vi "Read From Spreadsheet File (string)-Mod.vi"(0 "file path (dialog if empty)":path, 1 "format (%s)":string="%s", 5 "number of rows (all:-1)":i32=-1, 7 "max characters/row  (no limit:0)":i32, 9 "start of read offset (chars.:0)":i32, 11 "error in":errorcluster, 12 "transpose (no:F)":bool, 14 "delimiter (\\t)":string="\t") -> (3 "new file path (Not A Path if cancelled)":path, 4 "all rows":string[][](array[string]), 6 "first row":string[](array[string]), 8 "EOF?":bool, 10 "mark after read (chars.)":i32, 15 "error out":errorcluster)   [LabVIEW 2013]
doc: "Reads a specified number of lines or rows from a numeric text file beginning at a specified character offset and converts the data to a 2D, double-precision array of numbers, strings, or integers. You must manually select the polymorphic instance you want to use."
panel:
  in  "type (empty)":string[][](array[string])
  # "row\ncolumn"
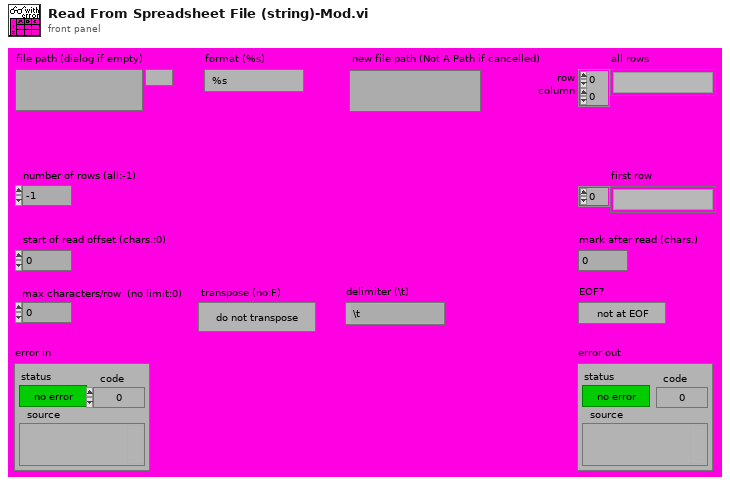
[diagram p1: front panel]
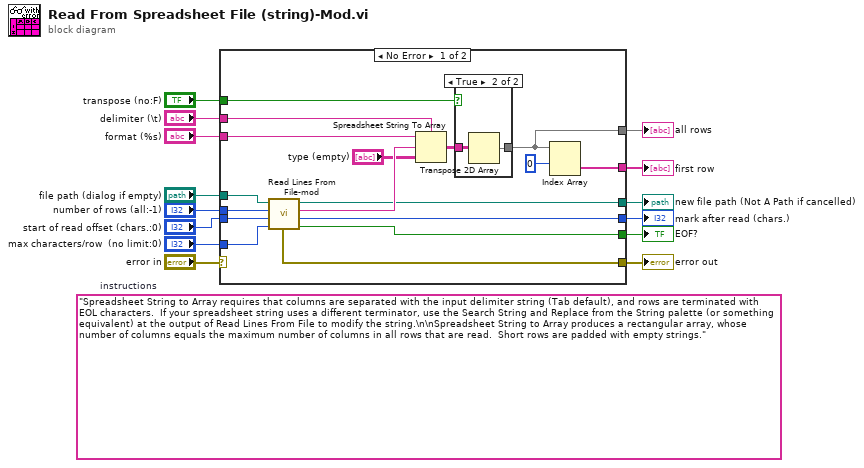
[diagram p0: block diagram]
diagram:
  (unwired) "Spreadsheet String to Array requires that columns are separated with the input delimiter string (Tab default), and rows are terminated with EOL characters.  If your spreadsheet string uses a different terminator, use the Search String and Replace from the String palette (or something equivalent) at the output of Read Lines From File to modify the string.\n\nSpreadsheet String to Array produces a rectangular array, whose number of columns equals the maximum number of columns in all rows that are read.  Short rows are padded with empty strings."  # instructions
  n1 = case shown="No Error" "error in" {
    selector: "error in" -> [_ w36]
    tunnel: "number of rows (all:-1)" -> [w31 _]
    tunnel: "file path (dialog if empty)" -> [w30 w35]
    tunnel: "max characters/row  (no limit:0)" -> [w29 _]
    tunnel: "start of read offset (chars.:0)" -> [w28 _]
    tunnel: "transpose (no:F)" -> [w26 _]
    tunnel: [w25 w35] -> w9
    tunnel: [w23 _] -> w8
    tunnel: "format (%s)" -> [w21 _]
    tunnel: "delimiter (\\t)" -> [w20 _]
    tunnel: [w19 _] -> w5
    tunnel: [w17 _] -> w4
    tunnel: [w16 _] -> w3
    tunnel: [w15 w36] -> w2
    frame No Error {
      n2 = call "Read Lines From File-mod.vi"("file path (dialog if empty)"=w30, "number of lines (all:-1)"=w31, "start of read offset (chars.:0)"=w28, "[max characters per line]  (no limit:0)"=w29) -> ("new file path (Not A Path if cancelled)"=w25:path, "line string"=w27:string, "mark after read (chars.)"=w23:i32, "EOF?"=w19:bool, "error out"=w15:errorcluster)  [unwired: 1 in]
      n3 = Spreadsheet String To Array(delimiter (Tab)=w20, format string=w21, spreadsheet string=w27, array type (2D Dbl)="type (empty)") -> (array=w18:string[][])
      n4 = case shown="True" w26 {
        tunnel: w18 -> [w32 w34]
        tunnel: [w32 w33] -> w16
        frame False {
        }
        frame True {
          n5 = Transpose 2D Array(2D array=w34) -> (transposed array=w33:string[][])
        }
      }
      n6 = Index Array(array=w16, index (row)=0) -> (element=w17:string[])  [unwired: 1 in]
    }
    frame Error {
    }
  }
  "new file path (Not A Path if cancelled)" <- w9
  "first row" <- w4
  "mark after read (chars.)" <- w8
  "all rows" <- w3
  "EOF?" <- w5
  "error out" <- w2
